vi "TSPopup.Get Control Value.vi"(7 "Prop Type":T1, 8 "error in (no error)":errorcluster, 11 "Control":refnum<vi>) -> (0 "error out":errorcluster, 2 "Value":variant, 3 "dup ref":refnum<vi>)   [LabVIEW 2013]
doc: "Returns the popup value as a variant. Reads from correct control in the popup cluster.\n\nType Sensitive Popup \nCopyright © 2007, J. David Saunders\nAll rights reserved."
uses:
  TSPopup.Data Type.ctl
panel:
  # "Type Sensitive Popup \nCopyright © 2007, J. David Saunders\nAll rights reserved."
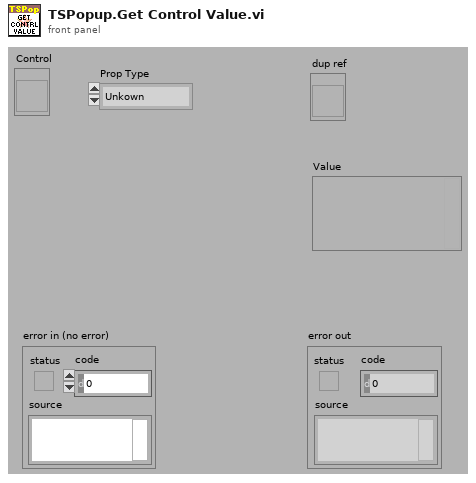
[diagram p1: front panel]
types:
  T1 = typedef "TSPopup.Data Type.ctl" = enum16{"Unkown", "NO POPUP", "String", "Integer", "Float", "Color", "Boolean", "Ring", "Captioned String", "Captioned Integer", "Button Color", "2 Int Cluster", "4 Int Cluster"}
  T2 = cluster{"left":i32, "top":i32, "right":i32, "bottom":i32}
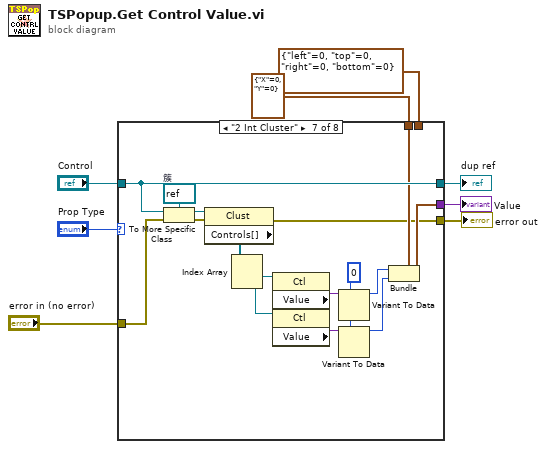
[diagram p0: block diagram]
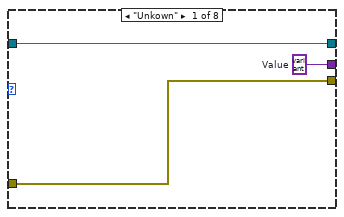
[diagram p2: hidden frame]
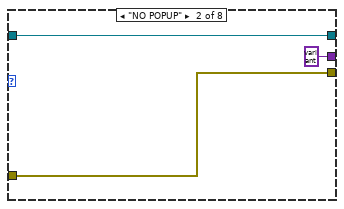
[diagram p3: hidden frame]
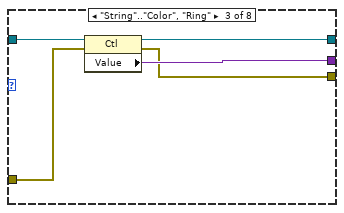
[diagram p4: hidden frame]
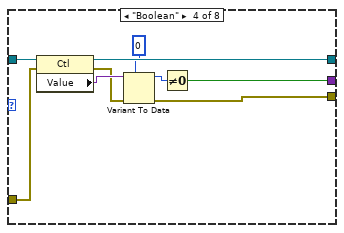
[diagram p5: hidden frame]
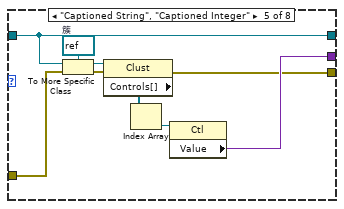
[diagram p6: hidden frame]
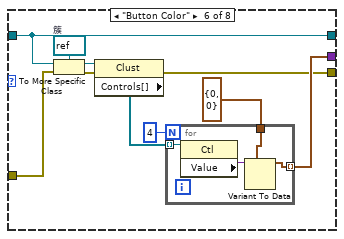
[diagram p7: hidden frame]
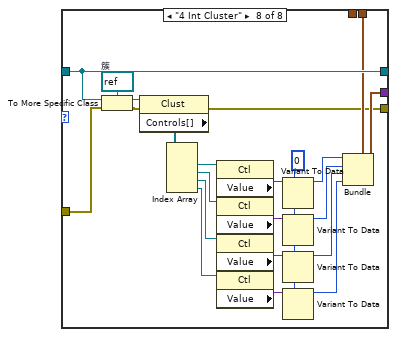
[diagram p8: hidden frame]
diagram:
  n1 = case shown="\"2 Int Cluster\"" "Prop Type" {
    tunnel: "Control" -> [w11 w14 w19 w28 w33 w42 w65 w87]
    tunnel: [w11 w14 w18 w27 w33 w42 w65 w87] -> w7
    tunnel: [w10 variant w17 w23 w32 w41 w55 w79] -> w3
    tunnel: cluster{"X":i32, "Y":i32} {"X"=0, "Y"=0} -> [_ _ _ _ _ _ w61 _]
    tunnel: T2 {"left"=0, "top"=0, "right"=0, "bottom"=0} ("rect") -> [_ _ _ _ _ _ _ w78]
    tunnel: "error in (no error)" -> [w9 w12 w16 w22 w31 w40 w54 w70]
    tunnel: [w9 w12 w15 w20 w29 w38 w52 w68] -> w1
    frame "Unkown" {
      w10 = variant  # Value
    }
    frame "NO POPUP" {
    }
    frame "String".."Color", "Ring" {
      n2 = property on="Property Node" class="Ctl"(reference=w19, error in=w16) -> (reference out=w18:refnum<vi>, error out=w15:errorcluster, "Value"=w17:variant)
    }
    frame "Boolean" {
      n3 = property on="Property Node" class="Ctl"(reference=w28, error in=w22) -> (reference out=w27:refnum<vi>, error out=w21:errorcluster, "Value"=w26:variant)
      n4 = Variant To Data(error in=w21, type=0, Variant=w26) -> (data=w24:i32, error out=w20:errorcluster)
      n5 = Not Equal To 0?(x=w24) -> (x != 0?=w23:bool)
    }
    frame "Captioned String", "Captioned Integer" {
      w34 = refnum<vi> refnum  # 簇
      n6 = To More Specific Class(target class=w34, reference=w33, error in=w31) -> (specific class reference=w35:refnum<vi>, error out=w30:errorcluster)
      n7 = property class="Clust"(reference=w35, error in=w30) -> (error out=w29:errorcluster, "Controls[]"=w36:refnum<vi>[])  [unwired: 1 out]
      n8 = Index Array(array=w36) -> (element=w37:refnum<vi>)  [unwired: 1 in]
      n9 = property class="Ctl"(reference=w37) -> ("Value"=w32:variant)  [unwired: 1 in, 2 out]
    }
    frame "Button Color" {
      w47 = refnum<vi> refnum  # 簇
      n10 = To More Specific Class(target class=w47, reference=w42, error in=w40) -> (specific class reference=w46:refnum<vi>, error out=w39:errorcluster)
      n11 = property class="Clust"(reference=w46, error in=w39) -> (error out=w38:errorcluster, "Controls[]"=w44:refnum<vi>[])  [unwired: 1 out]
      n12 = for {
        N: 4 -> [_]
        tunnel: w44 -> [w51] mode=indexing
        tunnel: cluster{u32, u32} {0, 0} -> [w49]
        tunnel: [w48] -> w41 mode=indexing
        n13 = property class="Ctl"(reference=w51) -> ("Value"=w50:variant)  [unwired: 1 in, 2 out]
        n14 = Variant To Data(type=w49, Variant=w50) -> (data=w48:cluster{u32, u32})  [unwired: 1 in, 1 out]
      }
    }
    frame "2 Int Cluster" {
      w58 = 0 ("x")
      w67 = refnum<vi> refnum  # 簇
      n15 = To More Specific Class(target class=w67, reference=w65, error in=w54) -> (specific class reference=w66:refnum<vi>, error out=w53:errorcluster)
      n16 = property class="Clust"(reference=w66, error in=w53) -> (error out=w52:errorcluster, "Controls[]"=w64:refnum<vi>[])  [unwired: 1 out]
      n17 = Index Array(array=w64) -> (element #1=w63:refnum<vi>, element #2=w62:refnum<vi>)  [unwired: 2 in]
      n18 = property class="Ctl"(reference=w63) -> ("Value"=w60:variant)  [unwired: 1 in, 2 out]
      n19 = property class="Ctl"(reference=w62) -> ("Value"=w59:variant)  [unwired: 1 in, 2 out]
      n20 = Variant To Data(type=w58, Variant=w60) -> (data=w56:i32)  [unwired: 1 in, 1 out]
      n21 = Variant To Data(type=w58, Variant=w59) -> (data=w57:i32)  [unwired: 1 in, 1 out]
      n22 = Bundle(cluster=w61, "X"=w56, "Y"=w57) -> (w55:cluster{"X":i32, "Y":i32})
    }
    frame "4 Int Cluster" {
      w73 = 0 ("x")
      w89 = refnum<vi> refnum  # 簇
      n23 = To More Specific Class(target class=w89, reference=w87, error in=w70) -> (specific class reference=w88:refnum<vi>, error out=w69:errorcluster)
      n24 = property class="Clust"(reference=w88, error in=w69) -> (error out=w68:errorcluster, "Controls[]"=w86:refnum<vi>[])  [unwired: 1 out]
      n25 = Index Array(array=w86) -> (element #1=w85:refnum<vi>, element #2=w84:refnum<vi>, element #3=w75:refnum<vi>, element #4=w74:refnum<vi>)  [unwired: 4 in]
      n26 = property class="Ctl"(reference=w85) -> ("Value"=w83:variant)  [unwired: 1 in, 2 out]
      n27 = property class="Ctl"(reference=w84) -> ("Value"=w82:variant)  [unwired: 1 in, 2 out]
      n28 = property class="Ctl"(reference=w75) -> ("Value"=w76:variant)  [unwired: 1 in, 2 out]
      n29 = property class="Ctl"(reference=w74) -> ("Value"=w77:variant)  [unwired: 1 in, 2 out]
      n30 = Variant To Data(type=w73, Variant=w83) -> (data=w80:i32)  [unwired: 1 in, 1 out]
      n31 = Variant To Data(type=w73, Variant=w82) -> (data=w81:i32)  [unwired: 1 in, 1 out]
      n32 = Variant To Data(type=w73, Variant=w76) -> (data=w72:i32)  [unwired: 1 in, 1 out]
      n33 = Variant To Data(type=w73, Variant=w77) -> (data=w71:i32)  [unwired: 1 in, 1 out]
      n34 = Bundle(cluster=w78, "left"=w80, "top"=w81, "right"=w72, "bottom"=w71) -> (w79:T2)
    }
  }
  "dup ref" <- w7
  "Value" <- w3
  "error out" <- w1
